vi "Init_Test.vi"(8 "error in (no error)":errorcluster caption="entrée d'erreur (pas d'erreur)", 11 "Delay en entrée":refnum<class "Reset_Variable_SIN.lvclass">) -> (0 "error out":errorcluster caption="sortie d'erreur", 3 "Delay en sortie":refnum<class "Reset_Variable_SIN.lvclass">)   [LabVIEW 2020, in "Library Test.lvlib" / "Reset_Variable_SIN.lvclass"]
uses:
  Reset_Variable_SIN.lvclass
  C:/Users/ngarcin/OneDrive - Altyor/Standard TB/Class/Test/Test (Default)/Test (Default).lvclass
  Commun VI/TypeDef/Commande Test/Commande Type Test.ctl
  Test_Without_Instr/Test_Without_Inst.lvclass
  Reset_Variable_SIN.lvclass/Reset_Variable_SIN.ctl
  Commun VI/Library Commun.lvlib
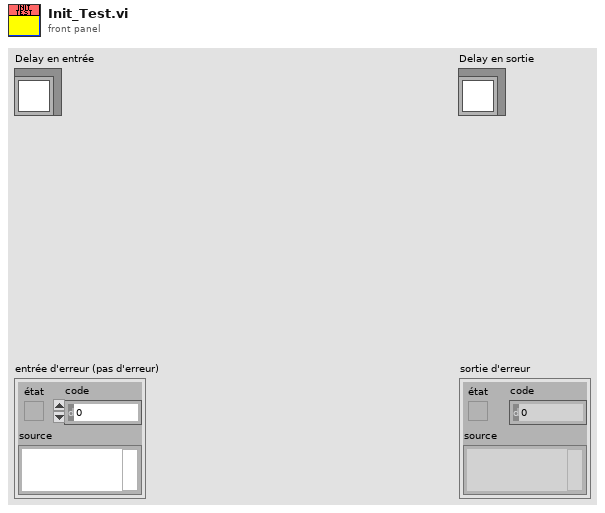
[diagram p1: front panel]
types:
  T1 = typedef "Library Commun.lvlib/Commande Type Test.ctl" = enum16{"Function", "Test", "Calculation"}
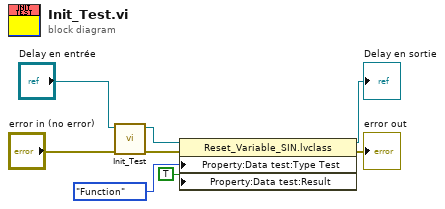
[diagram p0: block diagram]
diagram:
  n1 = call-parent "Init_Test.vi"("error in (no error)"="error in (no error)", "Test_Without_Inst en entrée"="Delay en entrée") -> ("error out"=w5:errorcluster, "Test_Without_Inst en sortie"=w6:refnum<class "Reset_Variable_SIN.lvclass">)  [unwired: 8 in]
  n2 = property class="Reset_Variable_SIN.lvclass"(reference=w6, error in=w5, "Property:Data test:Type Test"=Commande_Type_Test."Function" ("Type Test"), "Property:Data test:Result"=TRUE ("Result")) -> (reference out=→"Delay en sortie":refnum<class "Reset_Variable_SIN.lvclass">, error out=→"error out":errorcluster)
